vi "RSZVB Wait For OPC No Read.vi"(8 "error in (no error)":errorcluster {"code" format="%.0x"}, 9 "Timeout (300000 ms)":u32=300000, 10 "Command":string="*OPC?", 11 "VISA session":refnum<visa-resource-name>) -> (0 "error out":errorcluster {"code" format="%.0x"}, 3 "dup VISA session":refnum<visa-resource-name>)   [LabVIEW 2015]
doc: "This VI send a command to the instrument and waits for the response."
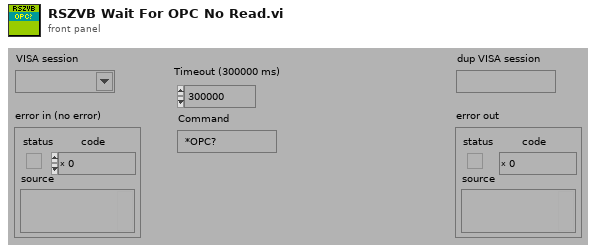
[diagram p1: front panel]
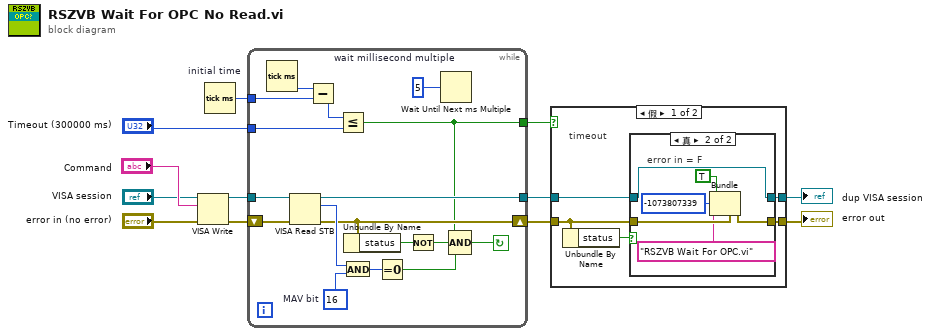
[diagram p0: block diagram]
diagram:
  n1 = VISA Write(VISA resource name="VISA session", write buffer="Command", error in (no error)="error in (no error)") -> (VISA resource name out=w3:refnum<visa-resource-name>, error out=w4:errorcluster)  [unwired: 1 out]
  n2 = Tick Count (ms) "initial time"() -> (millisecond timer value=w5:u32)
  n3 = while {
    tunnel: [w13] -> w6
    tunnel: w5 -> [w21]
    tunnel: "Timeout (300000 ms)" -> [w19]
    shift-left: w4 -> [w29]
    shift-right: [w18] -> w8
    tunnel: [w27] -> w7
    tunnel: w3 -> [w28]
    stop <- w15 continue-if-true
    w23 = u32 5  # wait millisecond multiple
    w25 = u16 16  # MAV bit
    n4 = Tick Count (ms)() -> (millisecond timer value=w22:u32)
    n5 = VISA Read STB(8:w29, 11:w28) -> (0:w18:errorcluster, 2:w26:u16, 3:w27:refnum<visa-resource-name>)
    n6 = Subtract(x=w22, y=w21) -> (x-y=w20:u32)
    n7 = Less Or Equal?(x=w20, y=w19) -> (x <= y?=w13:bool)
    n8 = And(x=w26, y=w25) -> (x .and. y?=w24:u16)
    n9 = Unbundle By Name(w18) -> ("status"=w17:bool)
    n10 = Equal To 0?(x=w24) -> (x = 0?=w14:bool)
    n11 = Not(x=w17) -> (.not. x?=w16:bool)
    n12 = Wait Until Next ms Multiple(millisecond multiple=w23) -> ()  [unwired: 1 out]
    n13 = Compound Arithmetic op=AND(w13, w16, w14) -> (w15:bool)
  }
  n14 = case shown="假" w6 {
    tunnel: w7 -> [w31 w44]
    tunnel: w8 -> [w33 w43]
    tunnel: [w32 w43] -> w11
    tunnel: [w30 w44] -> w10
    frame False {
      # "timeout"
      n15 = Unbundle By Name(w33) -> ("status"=w34:bool)
      n16 = case shown="真" w34 {
        tunnel: w33 -> [w36 w42]
        tunnel: [w36 w38] -> w32
        tunnel: w31 -> [w35 w37]
        tunnel: [w35 w37] -> w30
        frame False {
          # "error in = T"
        }
        frame True {
          # "error in = F"
          n17 = Bundle(cluster=w42, "status"=TRUE, "code"=-1073807339, "source"="RSZVB Wait For OPC.vi") -> (w38:errorcluster)
        }
      }
    }
    frame True {
      # "no timeout"
    }
  }
  "error out" <- w11
  "dup VISA session" <- w10
